vi "Simulation 4.vi"() -> ()   [LabVIEW 2024]
panel:
  out "A2P":bool(c317)
  out "Actuator Valve 2":bool
  out "A1P":bool(c317)
  in  "Actuator Valve 1":bool
  out "Multi-Segment Pipe 5":bool(c317)
  out "A2_pipe":bool(c317)
  out "A1_pipe":bool(c317)
  out "Multi-Segment Pipe 10":bool(c317)
  out "Multi-Segment Pipe 9":bool(c317)
  in  "stop":bool
  in  "Oil Pump":bool
  out "S2":bool
  out "S1":bool
  out "Tank 2":dbl(slide) scale=0.0..100.0
  out "Multi-Segment Pipe 7":bool(c317)
  out "Multi-Segment Pipe 6":bool(c317)
  out "Multi-Segment Pipe 4":bool(c317)
  out "Multi-Segment Pipe 3":bool(c317)
  out "Multi-Segment Pipe 2":bool(c317)
  out "Tank 1":dbl(slide) scale=0.0..100.0
  # "Level Sensor"
  # "Oil Source"
  # "Level Sensor"
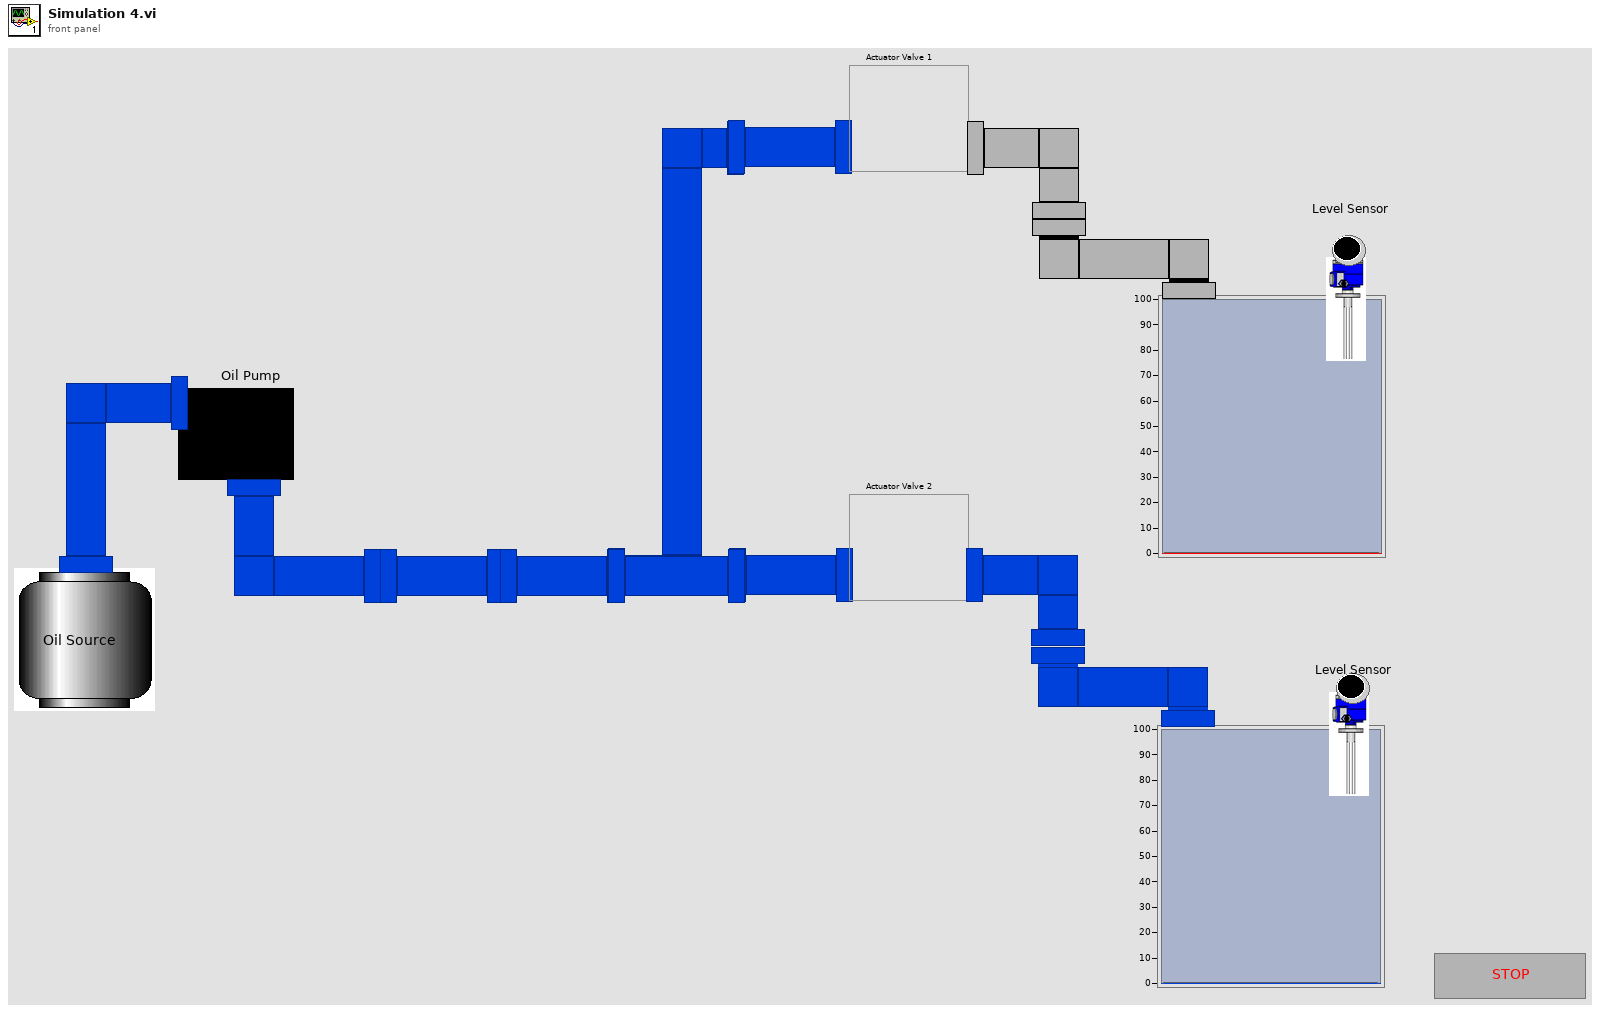
[diagram p1: front panel]
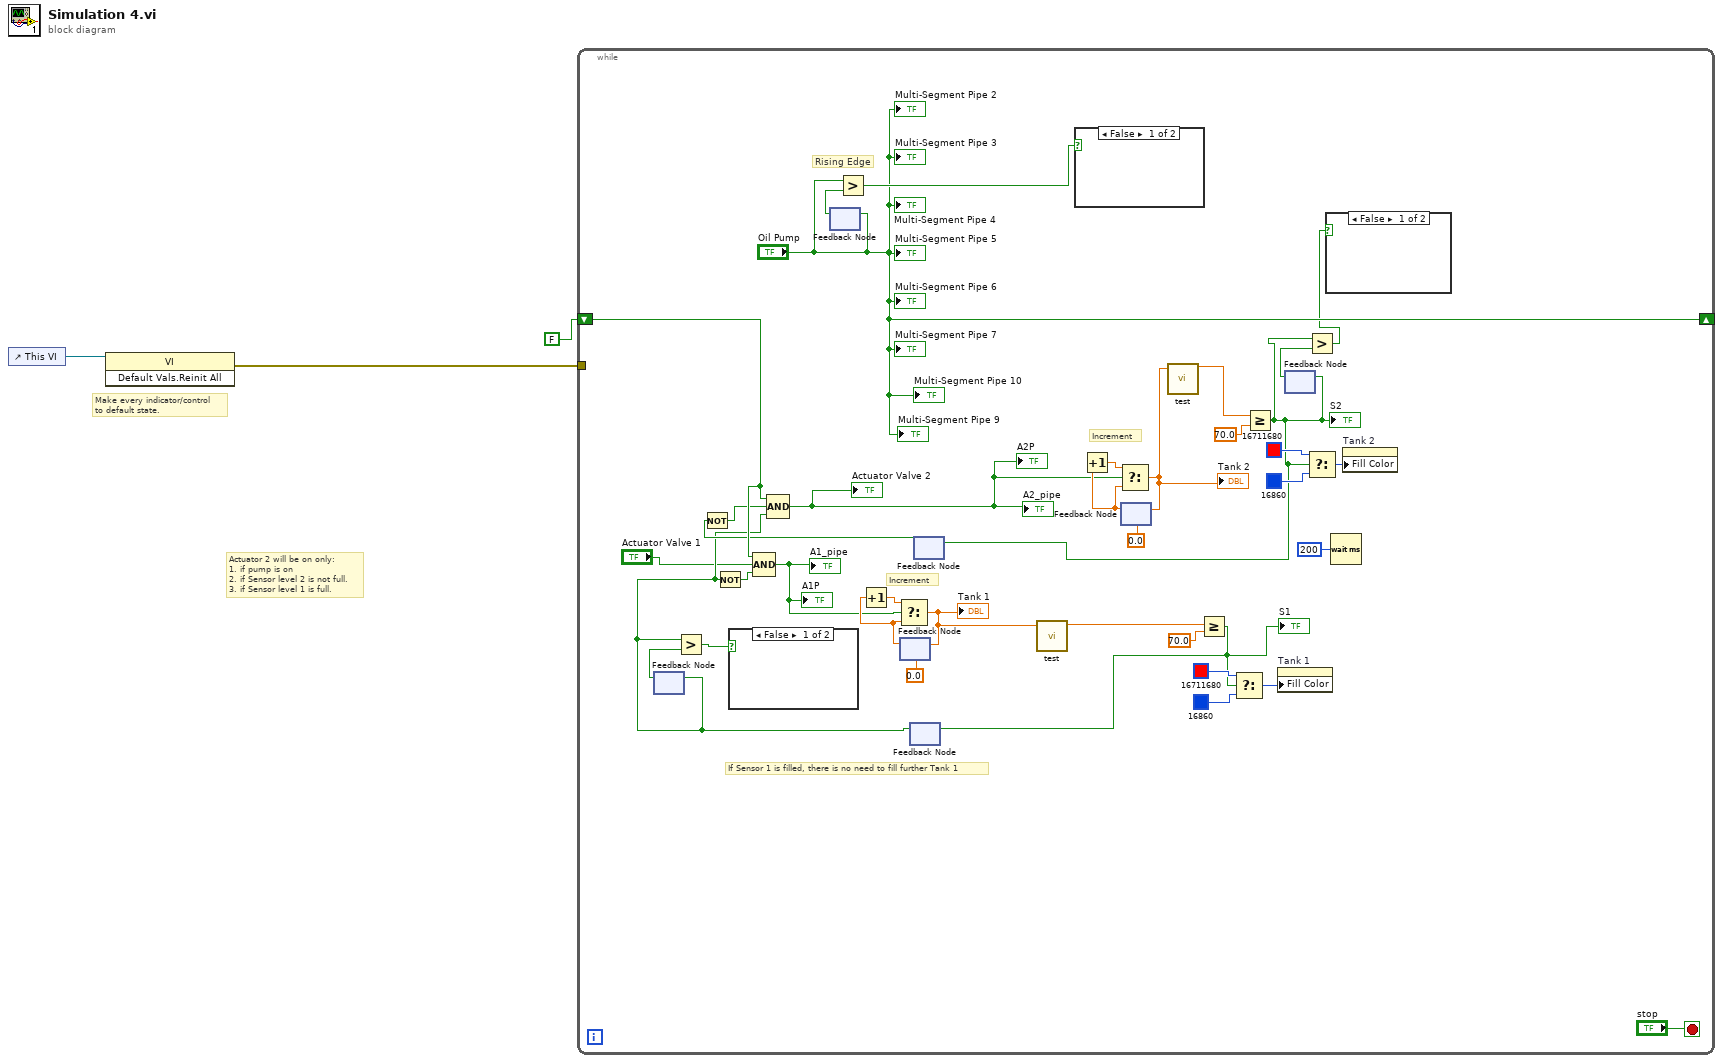
[diagram p0: block diagram]
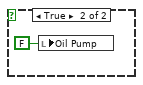
[diagram p2: hidden frame]
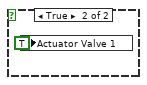
[diagram p3: hidden frame]
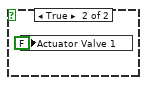
[diagram p4: hidden frame]
diagram:
  # "Actuator 2 will be on only:\n1. if pump is on\n2. if Sensor level 2 is not full.\n3. if Sensor level 1 is full."
  # "Make every indicator/control\nto default state."
  n1 = control-ref of="This VI"() -> (w2:refnum<vi>)
  n2 = invoke class="VI" method="Default Vals.Reinit All"(reference=w2) -> (error out=w1:errorcluster)  [unwired: 2 in, 2 out]
  n3 = while {
    shift-right: ["Oil Pump"] -> _
    shift-left: FALSE -> [w39]
    tunnel: w1 -> [_]
    stop <- "stop" stop-if-true
    # "Increment"
    # "Increment"
    # "If Sensor 1 is filled, there is no need to fill further Tank 1"
    # "Rising Edge"
    n4 = feedback #1() -> (w22:bool)  [unwired: 1 in]
    n5 = feedback #2() -> (w16:bool)  [unwired: 1 in]
    n6 = feedback-in #2("Oil Pump") -> ()
    n7 = Greater?(x="Oil Pump", y=w16) -> (0:w15:bool)
    n8 = feedback #3(0.0) -> (w34:dbl)
    n9 = Increment(x=w34) -> (x+1=w33:dbl)
    n10 = feedback #4() -> (w17:bool)  [unwired: 1 in]
    n11 = feedback-in #1(w17) -> ()
    n12 = Greater?(x=w17, y=w22) -> (0:w21:bool)
    n13 = Not(x=w17) -> (.not. x?=w20:bool)
    n14 = case shown="False" w21 {
      frame False {
      }
      frame True {
        n15 = local write "Actuator Valve 1"(FALSE ("Actuator 1")) -> ()
      }
    }
    n16 = Compound Arithmetic op=AND(w39, "Actuator Valve 1", w20) -> (w10:bool)
    "A1_pipe" <- w10
    "A1P" <- w10
    n17 = Select(t=w33, s=w10, f=w34) -> (s? t:f=w6:dbl)
    "Tank 1" <- w6
    n18 = feedback-in #3(w6) -> ()
    n19 = feedback #5() -> (w19:bool)  [unwired: 1 in]
    n20 = Not(x=w19) -> (.not. x?=w18:bool)
    n21 = Compound Arithmetic op=AND(w39, w18, w17) -> (w8:bool)
    "A2_pipe" <- w8
    "Actuator Valve 2" <- w8
    "A2P" <- w8
    n22 = call "test.vi"("invalue"=w6) -> ("characters"=w7:dbl)  [unwired: 10 in]
    n23 = case shown="False" w15 {
      frame False {
      }
      frame True {
        n24 = local write "Actuator Valve 1"(TRUE ("Actuator 1")) -> ()
      }
    }
    n25 = feedback #6(0.0) -> (w35:dbl)
    n26 = Increment(x=w35) -> (x+1=w36:dbl)
    n27 = Select(t=w36, s=w8, f=w35) -> (s? t:f=w4:dbl)
    "Tank 2" <- w4
    n28 = feedback-in #6(w4) -> ()
    n29 = call "test.vi"("invalue"=w4) -> ("characters"=w5:dbl)  [unwired: 10 in]
    n30 = Greater Or Equal?(x=w7, y=70.0) -> (x >= y?=w23:bool)
    "S1" <- w23
    n31 = feedback-in #4(w23) -> ()
    n32 = Select(t=u32 16711680 ("Fill Color"), s=w23, f=u32 16860 ("Fill Color")) -> (s? t:f=w24:u32)
    n33 = Greater Or Equal?(x=w5, y=70.0) -> (x >= y?=w13:bool)
    "S2" <- w13
    n34 = feedback-in #5(w13) -> ()
    n35 = property on="Tank 1" class="Slide (strict)"("Fill Color"=w24) -> ()  [unwired: 2 in, 2 out]
    n36 = feedback #7() -> (w12:bool)  [unwired: 1 in]
    n37 = feedback-in #7(w13) -> ()
    n38 = Greater?(x=w13, y=w12) -> (0:w11:bool)
    n39 = Select(t=u32 16711680 ("Fill Color"), s=w13, f=u32 16860 ("Fill Color")) -> (s? t:f=w28:u32)
    n40 = case shown="False" w11 {
      frame False {
      }
      frame True {
        n41 = local write "Oil Pump"(FALSE ("Actuator 1")) -> ()
      }
    }
    n42 = Wait (ms)(milliseconds to wait=u32 200) -> ()  [unwired: 1 out]
    n43 = property on="Tank 2" class="Slide (strict)"("Fill Color"=w28) -> ()  [unwired: 2 in, 2 out]
    "Multi-Segment Pipe 2" <- "Oil Pump"
    "Multi-Segment Pipe 3" <- "Oil Pump"
    "Multi-Segment Pipe 4" <- "Oil Pump"
    "Multi-Segment Pipe 5" <- "Oil Pump"
    "Multi-Segment Pipe 6" <- "Oil Pump"
    "Multi-Segment Pipe 7" <- "Oil Pump"
    "Multi-Segment Pipe 9" <- "Oil Pump"
    "Multi-Segment Pipe 10" <- "Oil Pump"
  }
